vi "main.vi"() -> ()   [LabVIEW 2015]
panel:
  in  "Axe":i32=1
  in  "Deceleration":dbl
  in  "Acceleration":dbl
  in  "Vitesse":dbl
  in  "Angle":dbl
  out "Sequence":T1
  in  "Enregistrer sequence X":bool
  in  "Vitesse Manuelle Y":dbl
  in  "Vitesse Manuelle X":dbl
  in  "Decel":dbl
  in  "Accel":dbl
  in  "Ressolution Codeur":dbl
  in  "Diametre Galet Codeur":dbl
  in  "Diametre Plateau":dbl
  in  "Decel Max":dbl
  in  "Accel Max":dbl
  in  "Vitesse Max":dbl
  in  "PARAM DLG":bool
  in  "stop moteurs":bool
  in  "Go2":bool
  in  "Go1":bool
  in  "Vitesse Y":dbl
  in  "Vitesse X":dbl
  in  "Angle Y":dbl
  in  "Angle X":dbl
  in  "Remise a zero Y":bool
  in  "Remise a zero X":bool
  in  "stop":bool
  in  "x+":bool
  in  "x-":bool
  in  "y+":bool
  in  "y-":bool
  in  "x+y+":bool
  in  "x-y+":bool
  in  "x-y-":bool
  in  "x+y-":bool
  out "Deverouillé":bool
  out "Connecté":bool
  # "Control Manuel Y"
  # "Deplacement Automatique"
  # "Control Manuel X"
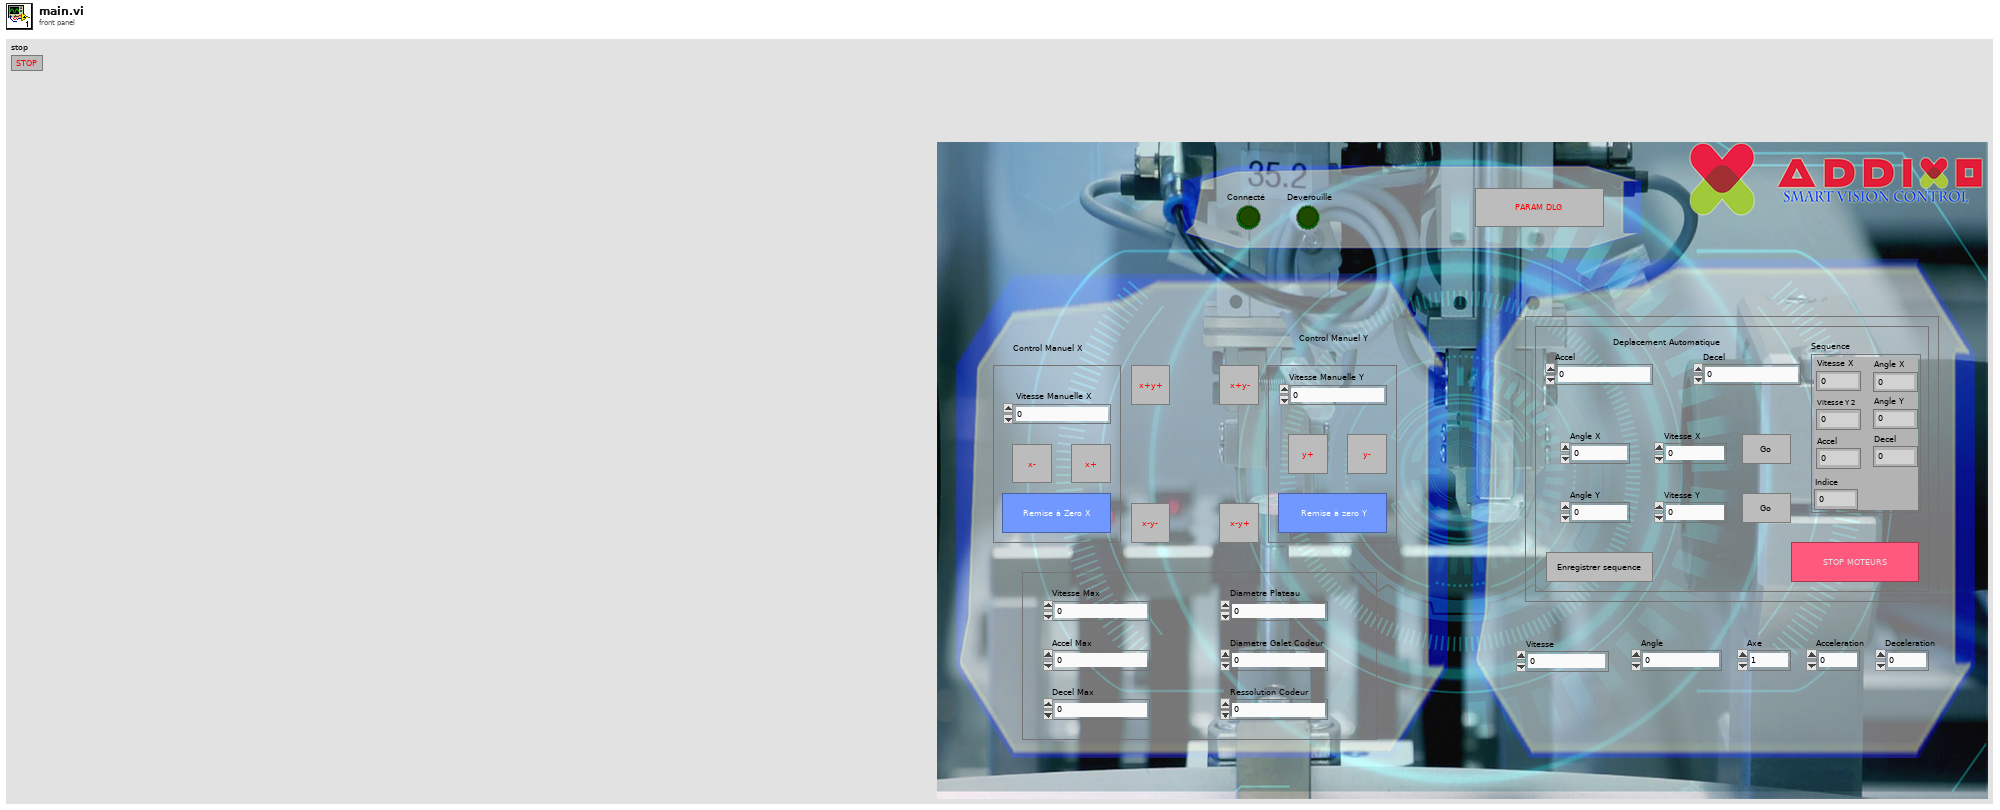
[diagram p1: front panel]
types:
  T1 = cluster{"Angle X":dbl, "Vitesse X":dbl, "Angle Y":dbl, "Accel":dbl, "Decel":dbl, "Indice":dbl, "Vitesse Y 2":dbl}
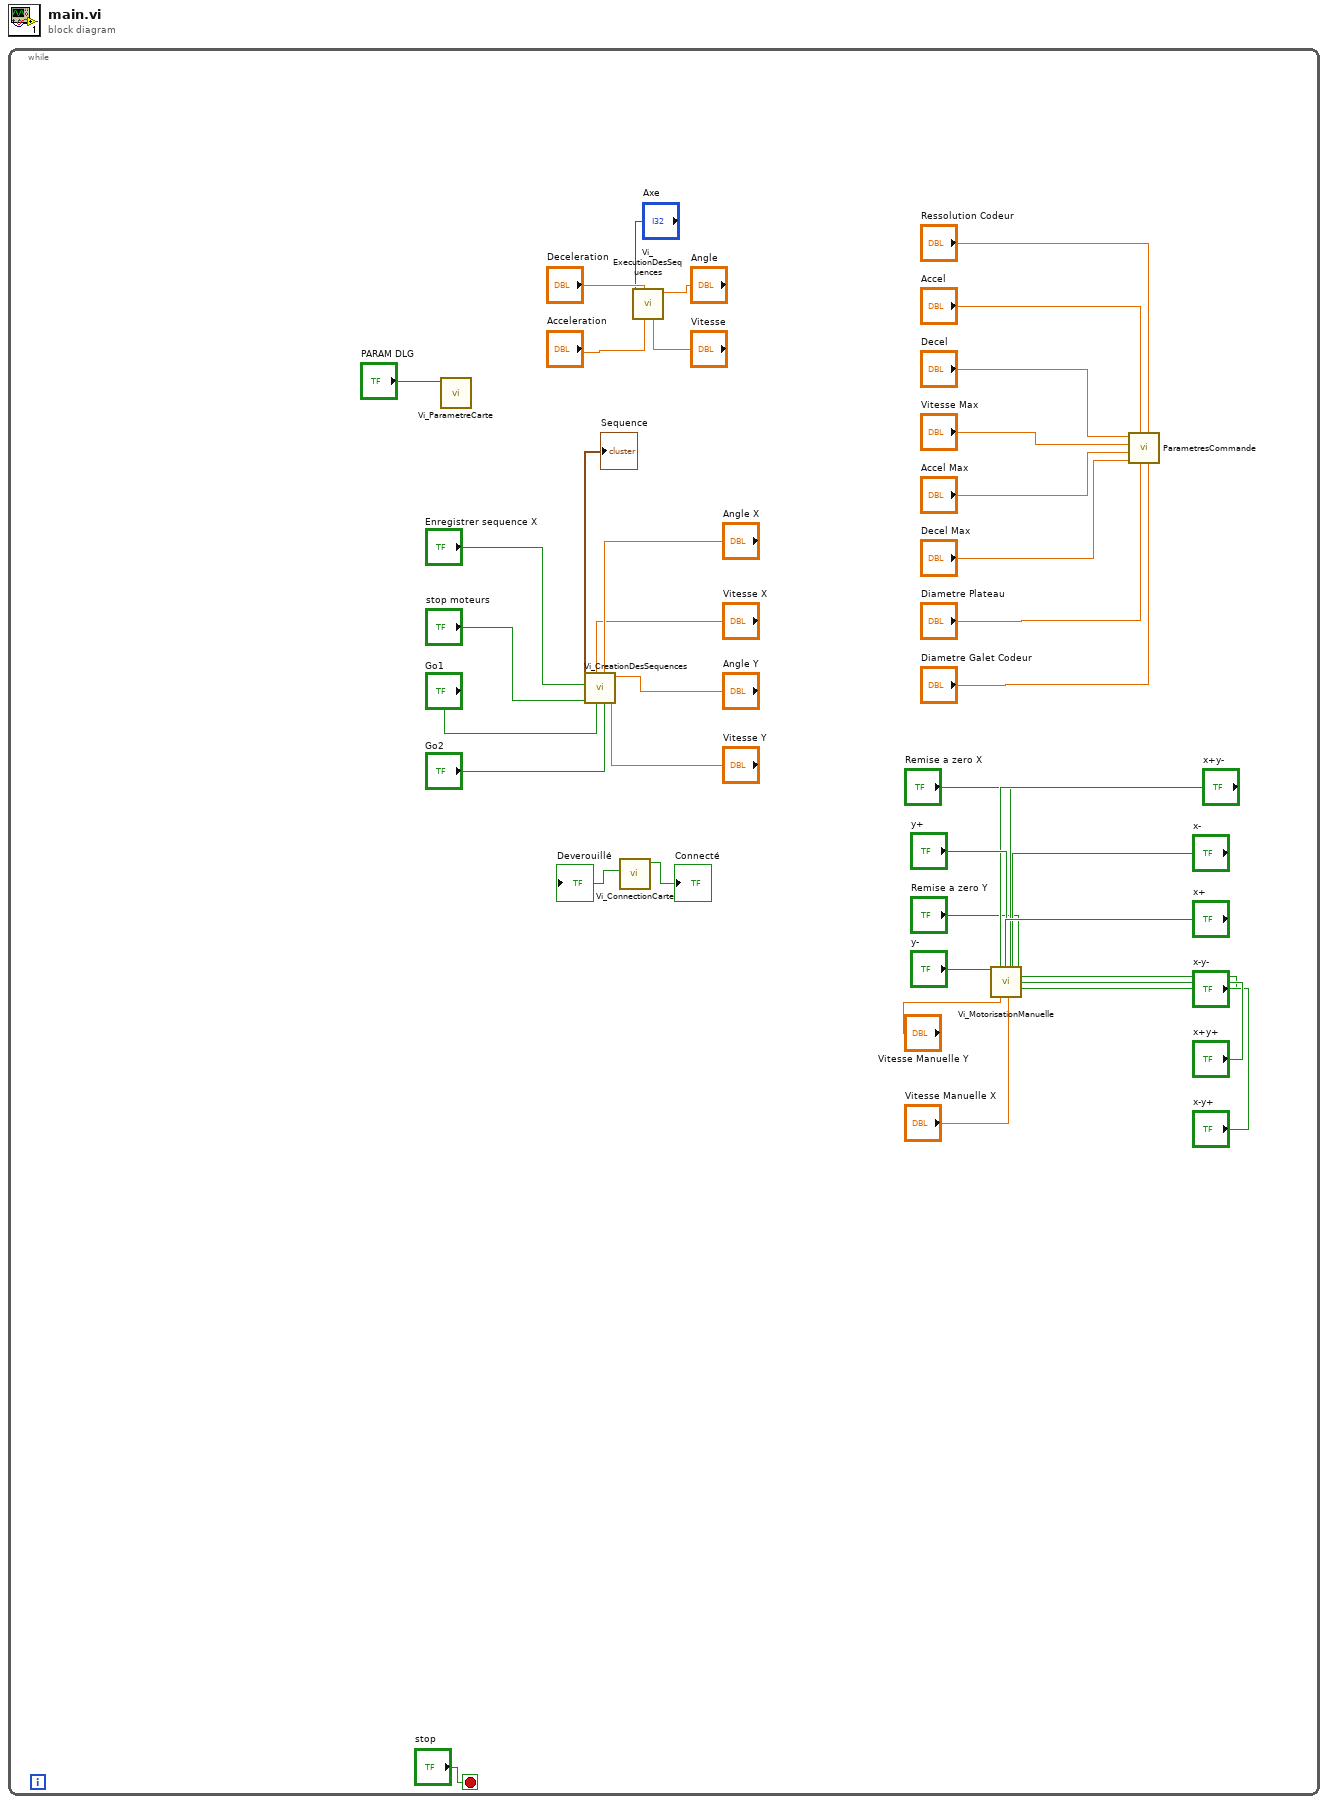
[diagram p0: block diagram]
diagram:
  n1 = while {
    stop <- "stop" stop-if-true
    n2 = call "Vi_ParametreCarte.vi"("PARAM DLG"="PARAM DLG") -> ()  [unwired: 9 in, 2 out]
    n3 = call "Vi_CreationDesSequences.vi"("Go2"="Go2", "Angle X"="Angle X", "Go1"="Go1", "Vitesse X"="Vitesse X", "stop moteurs"="stop moteurs", "Vitesse Y"="Vitesse Y", "Enregistrer sequence X"="Enregistrer sequence X", "Angle Y"="Angle Y") -> ("Sequence"=→"Sequence":T1)  [unwired: 1 in, 2 out]
    n4 = call "Vi_ConnectionCarte.vi"() -> ("Deverouillé"=→"Deverouillé":bool, "Connecté"=→"Connecté":bool)  [unwired: 10 in]
    n5 = call "Vi_ExecutionDesSequences.vi"("Acceleration"="Acceleration", "Deceleration"="Deceleration", "Axe"="Axe", "Vitesse"="Vitesse", "Angle"="Angle") -> ()  [unwired: 5 in, 2 out]
    n6 = call "Vi_MotorisationManuelle.vi"("x+"="x+", "Vitesse Manuelle Y"="Vitesse Manuelle Y", "Vitesse Manuelle X"="Vitesse Manuelle X", "x-"="x-", 5:"x-y-", "x+y+"="x+y+", "x-y+"="x-y+", "Remise a zero X"="Remise a zero X", "x+y-"="x+y-", "y+"="y+", 14:"y-", "Remise a zero Y"="Remise a zero Y") -> ()  [unwired: 2 in, 2 out]
    n7 = call "ParametresCommande.vi"("Diametre Galet Codeur"="Diametre Galet Codeur", "Ressolution Codeur"="Ressolution Codeur", "Diametre Plateau"="Diametre Plateau", "Accel"="Accel", "Decel Max"="Decel Max", "Accel Max"="Accel Max", "Vitesse Max"="Vitesse Max", "Decel"="Decel") -> ()  [unwired: 4 in]
  }
